vi "VAJ velocity in timing count.vi"(8 "dt":dbl, 9 "time":dbl, 11 "Array":cluster{"Numeric":dbl, "Numeric":dbl}[](array[cluster])) -> (0 "t4?":bool, 2 "velocity":dbl, 4 "finish":bool)   [LabVIEW 2019]
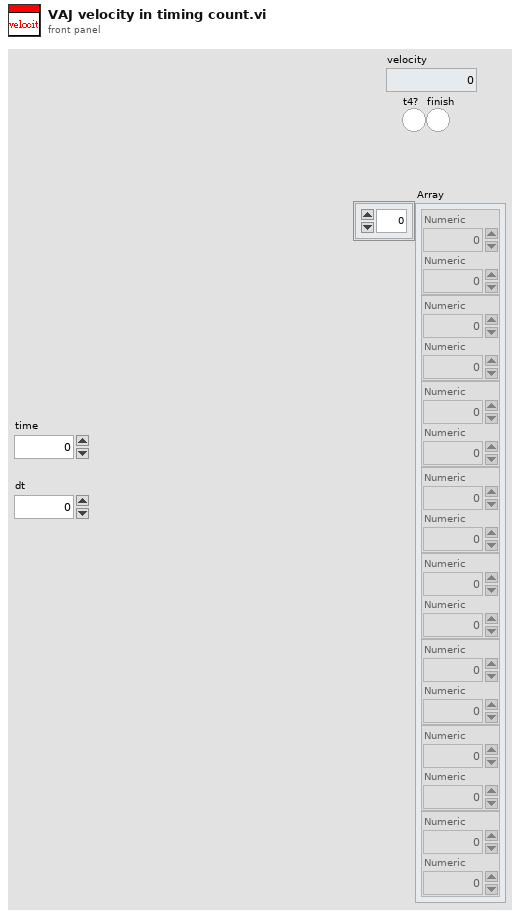
[diagram p1: front panel]
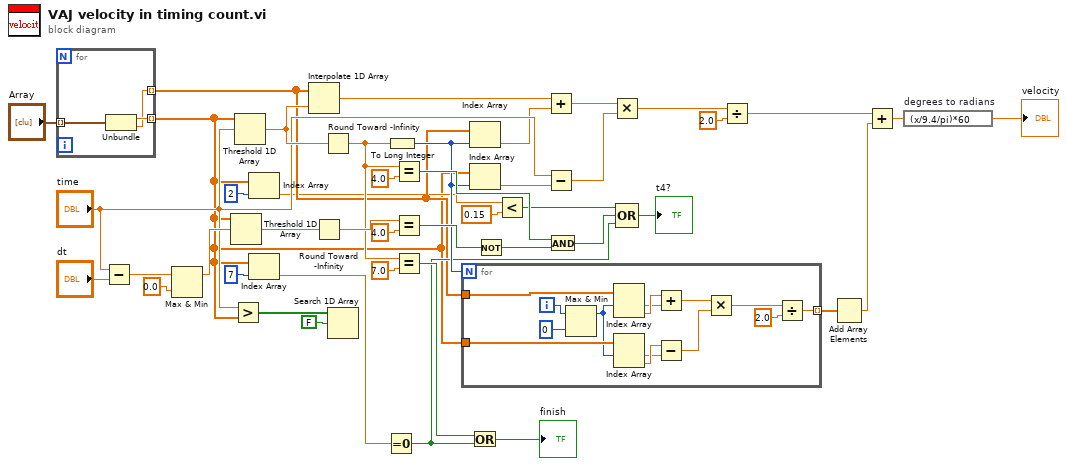
[diagram p0: block diagram]
diagram:
  n1 = for {
    tunnel: "Array" -> [w47] mode=indexing
    tunnel: [w46] -> w1 mode=indexing
    tunnel: [w45] -> w6 mode=indexing
    n2 = Unbundle(w47) -> ("Numeric"=w46:dbl, "Numeric"=w45:dbl)
  }
  n3 = Subtract(x="time", y="dt") -> (x-y=w33:dbl)
  n4 = Max & Min(x=w33, y=0.0) -> (max(x,y)=w22:dbl)  [unwired: 1 out]
  n5 = Threshold 1D Array(2:w22, 3:w1) -> (0:w32:dbl)  [unwired: 1 in]
  n6 = Greater?(x="time", y=w1) -> (0:w43:bool[])
  n7 = Threshold 1D Array(2:"time", 3:w1) -> (0:w20:dbl)  [unwired: 1 in]
  n8 = Index Array(array=w1, index=2) -> (element=w4:dbl)
  n9 = Index Array(array=w1, index=7) -> (element=w8:dbl)
  n10 = Interpolate 1D Array(1:w20, 2:w6) -> (0:w16:dbl)
  n11 = Round Toward -Infinity(1:w32) -> (0:w25:dbl)
  n12 = Round Toward -Infinity(1:w20) -> (0:w18:dbl)
  n13 = Search 1D Array(1D array=w43, element=FALSE) -> ()  [unwired: 1 in, 1 out]
  n14 = Equal To 0?(x=w8) -> (x = 0?=w7:bool)
  n15 = To Long Integer(number=w18) -> (32bit integer=w17:i32)
  n16 = Equal?(x=w18, y=4.0) -> (x = y?=w28:bool)
  n17 = Equal?(x=w25, y=4.0) -> (x = y?=w29:bool)
  n18 = Equal?(x=w18, y=7.0) -> (x = y?=w23:bool)
  n19 = for {
    N: w17 -> [_]
    tunnel: w6 -> [w61]
    tunnel: w1 -> [w58]
    tunnel: [w51] -> w41 mode=indexing
    i -> [w48]
    n20 = Max & Min(x=w48, y=0) -> (max(x,y)=w49:i32)  [unwired: 1 out]
    n21 = Index Array(array=w61, index #1=w49) -> (element #1=w59:dbl, element #2=w60:dbl)  [unwired: 1 in]
    n22 = Index Array(array=w58, index #1=w49) -> (element #1=w56:dbl, element #2=w57:dbl)  [unwired: 1 in]
    n23 = Add(x=w60, y=w59) -> (x+y=w55:dbl)
    n24 = Subtract(x=w57, y=w56) -> (x-y=w54:dbl)
    n25 = Multiply(x=w55, y=w54) -> (x*y=w53:dbl)
    n26 = Divide(x=w53, y=2.0) -> (x/y=w51:dbl)
  }
  n27 = Index Array(array=w6, index=w17) -> (element=w15:dbl)
  n28 = Index Array(array=w1, index=w17) -> (element=w39:dbl)
  n29 = Or(x=w23, y=w7) -> (x .or. y?=→"finish":bool)
  n30 = Not(x=w29) -> (.not. x?=w27:bool)
  n31 = Less?(x=w4, y=0.15) -> (x < y?=w2:bool)
  n32 = Add(x=w16, y=w15) -> (x+y=w14:dbl)
  n33 = Subtract(x="time", y=w39) -> (x-y=w38:dbl)
  n34 = And(x=w28, y=w27) -> (x .and. y?=w26:bool)
  n35 = Multiply(x=w14, y=w38) -> (x*y=w37:dbl)
  n36 = Compound Arithmetic op=OR(w2, w26, w7) -> (→"t4?":bool)
  n37 = Divide(x=w37, y=2.0) -> (x/y=w35:dbl)
  n38 = Add Array Elements(numeric array=w41) -> (sum=w40:dbl)
  n39 = Add(x=w35, y=w40) -> (x+y=w12:dbl)
  n40 = expression code="(x/9.4/pi)*60" "degrees to radians"(w12) -> (→"velocity":dbl)
